vi "Handle Tables after row deletion.vi"(0 "table.Data":string[][](array[string]), 5 "table.Stats":string[][](array[string]), 7 "DataRowIndex":i32, 9 "StatRowIndex":i32, 11 "StateCalled":string) -> ()   [LabVIEW 2013]
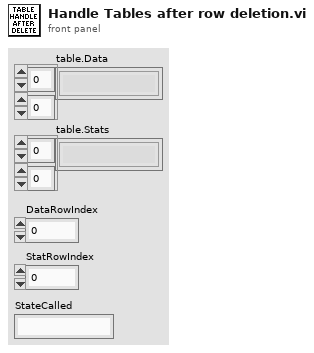
[diagram p1: front panel]
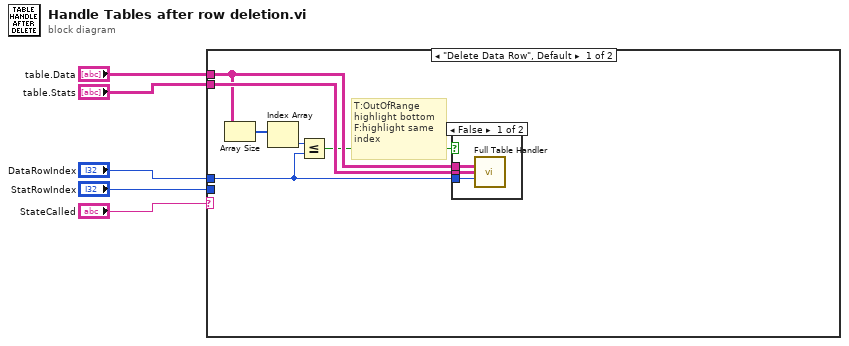
[diagram p0: block diagram]
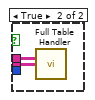
[diagram p2: hidden frame]
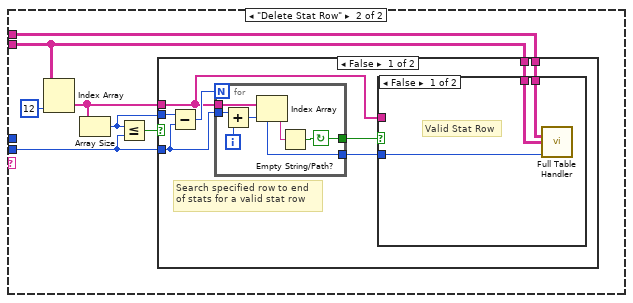
[diagram p3: hidden frame]
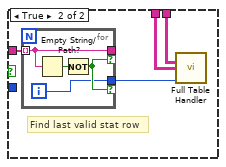
[diagram p4: hidden frame]
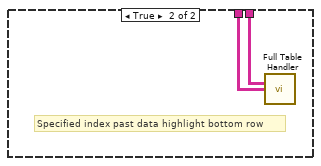
[diagram p5: hidden frame]
diagram:
  n1 = case shown="\"Delete Data Row\", Default" "StateCalled" {
    tunnel: "DataRowIndex" -> [w7 _]
    tunnel: "StatRowIndex" -> [_ w22]
    tunnel: "table.Stats" -> [w11 w20]
    tunnel: "table.Data" -> [w10 w23]
    frame "Delete Data Row", Default {
      # "T:OutOfRange\nhighlight bottom\nF:highlight same\nindex"
      n2 = Array Size(array=w10) -> (size(s)=w9:i32[])
      n3 = Index Array(array=w9) -> (element=w8:i32)  [unwired: 1 in]
      n4 = Less Or Equal?(x=w8, y=w7) -> (x <= y?=w6:bool)
      n5 = case shown="False" w6 {
        tunnel: w11 -> [w13 w16]
        tunnel: w10 -> [w14 w15]
        tunnel: w7 -> [w12 _]
        frame False {
          n6 = call "Full Table Handler.vi"("table.Data"=w14, "table.Stats"=w13, "Data Row Index"=w12) -> ()  [unwired: 13 in]
        }
        frame True {
          n7 = call "Full Table Handler.vi"("table.Data"=w15, "table.Stats"=w16) -> ()  [unwired: 14 in]
        }
      }
    }
    frame "Delete Stat Row" {
      n8 = Index Array(array=w20, index (col)=12 ("disabled index (col)")) -> (element=w18:string[])  [unwired: 1 in]
      n9 = Array Size(array=w18) -> (size(s)=w17:i32)
      n10 = Less Or Equal?(x=w17, y=w22) -> (x <= y?=w21:bool)
      n11 = case shown="False" w21 {
        tunnel: w23 -> [w26 w50]
        tunnel: w22 -> [w29 _]
        tunnel: w20 -> [w25 w49]
        tunnel: w18 -> [w24 _]
        tunnel: w17 -> [w31 _]
        frame False {
          # "Search specified row to end\nof stats for a valid stat row"
          n12 = Subtract(x=w31, y=w29) -> (x-y=w30:i32)
          n13 = for {
            N: w30 -> [_]
            tunnel: w24 -> [w48]
            tunnel: w29 -> [w47]
            tunnel: [w44] -> w28
            tunnel: [w43] -> w27
            i -> [w46]
            stop <- w44 continue-if-true
            n14 = Add(x=w47, y=w46) -> (x+y=w43:i32)
            n15 = Index Array(array=w48, index=w43) -> (element=w45:string)
            n16 = Empty String/Path?(string/path=w45) -> (empty?=w44:bool)
          }
          n17 = case shown="False" w28 {
            tunnel: w27 -> [w34 _]
            tunnel: w24 -> [_ w38]
            tunnel: w26 -> [w33 w36]
            tunnel: w25 -> [w32 w35]
            frame False {
              # "Valid Stat Row"
              n18 = call "Full Table Handler.vi"("table.Data"=w33, "table.Stats"=w32, "Stat Row Index"=w34) -> ()  [unwired: 13 in]
            }
            frame True {
              # "Find last valid stat row"
              n19 = for {
                tunnel: w38 -> [w42] mode=indexing
                tunnel: [w42] -> _ if=w40
                tunnel: [w39] -> w37 if=w40
                i -> [w39]
                n20 = Empty String/Path?(string/path=w42) -> (empty?=w41:bool)
                n21 = Not(x=w41) -> (.not. x?=w40:bool)
              }
              n22 = call "Full Table Handler.vi"("table.Data"=w36, "table.Stats"=w35, "Stat Row Index"=w37) -> ()  [unwired: 13 in]
            }
          }
        }
        frame True {
          # "Specified index past data highlight bottom row"
          n23 = call "Full Table Handler.vi"("table.Data"=w50, "table.Stats"=w49) -> ()  [unwired: 14 in]
        }
      }
    }
  }
